vi "p1.vi"() -> ()   [LabVIEW 2025, in "d3.lvlib"]
uses:
  d3.lvlib
  AOC/AOC.lvlib
  <userlib>/_OpenG.lib/string/string.llb/openg_string.lvlib
panel:
  in  "Example":string="987654321111111\n811111111111119\n234234234234278\n818181911112111"
  in  "Example":bool
  out "Answer":i64=7746
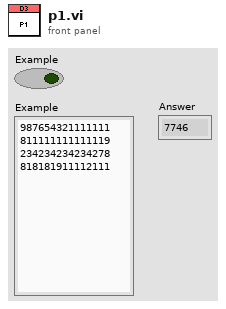
[diagram p1: front panel]
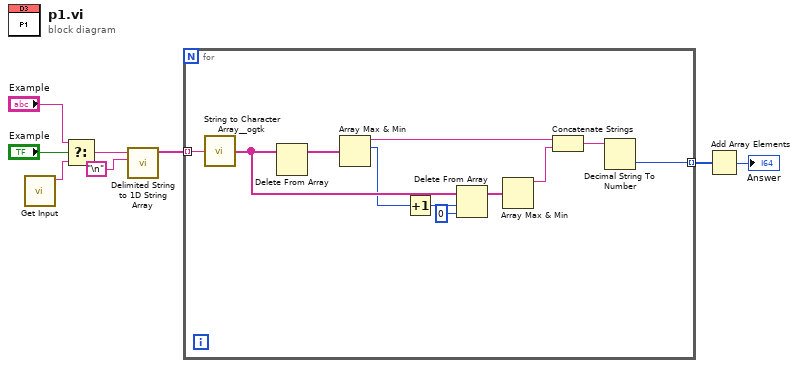
[diagram p0: block diagram]
diagram:
  n1 = call "Get Input.vi"() -> ("Input"=w8:string)  [unwired: 11 in]
  n2 = Select(t="Example", s="Example", f=w8) -> (s? t:f=w5:string)
  n3 = call <vilib>:"Delimited String to 1D String Array.vi"("delimiter"="\n", "delimited string"=w5) -> ("string array"=w3:string[])  [unwired: 9 in]
  n4 = for {
    tunnel: w3 -> [w19] mode=indexing
    tunnel: [w12] -> w2 mode=indexing
    n5 = call <userlib>:"String to Character Array__ogtk.vi"("Input String"=w19) -> ("Character Array"=w17:string[])
    n6 = Delete From Array(array=w17) -> (array with subset deleted=w18:string[])  [unwired: 2 in, 1 out]
    n7 = Array Max & Min(array=w18) -> (max value=w14:string, max index (indices)=w11:i32)  [unwired: 2 out]
    n8 = Increment(x=w11) -> (x+1=w10:i32)
    n9 = Delete From Array(array=w17, length=w10, index=0) -> (array with subset deleted=w16:string[])  [unwired: 1 out]
    n10 = Array Max & Min(array=w16) -> (max value=w15:string)  [unwired: 3 out]
    n11 = Concatenate Strings(w14, w15) -> (w13:string)
    n12 = Decimal String To Number(string=w13) -> (number=w12:i32)  [unwired: 2 in, 1 out]
  }
  n13 = Add Array Elements(numeric array=w2) -> (sum=→"Answer":i32)
